vi "Main.vi"() -> ()   [LabVIEW 2015]
uses:
  TypeDefs/Queue Data.ctl
  FGV/Timer Actions.ctl
  SubVIs/App Data.vi
  SubVIs/App Strings.vi
panel:
  in  "Period [s]":dbl
  in  "Device name":tag="myDAQ1"
  out "Time Elapsed":dbl format="%<%M:%S>t"
  out "Status":string
  in  "Time [ms]":dbl
  in  "Frequency":dbl
  in  "Stop Button":bool
  in  "Acquire Button":bool
  out "Waveform Graph":dbl[](graph)
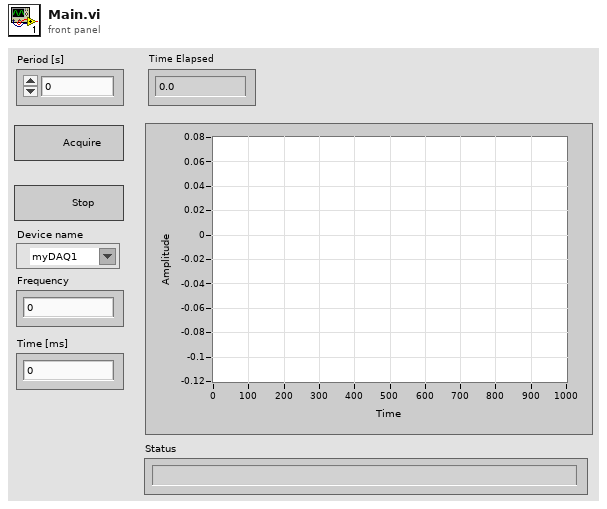
[diagram p1: front panel]
types:
  T1 = typedef "Timer Actions.ctl" = enum16{"Reset", "Get"}
  T2 = typedef "Queue Data.ctl" = cluster{"Action":string}
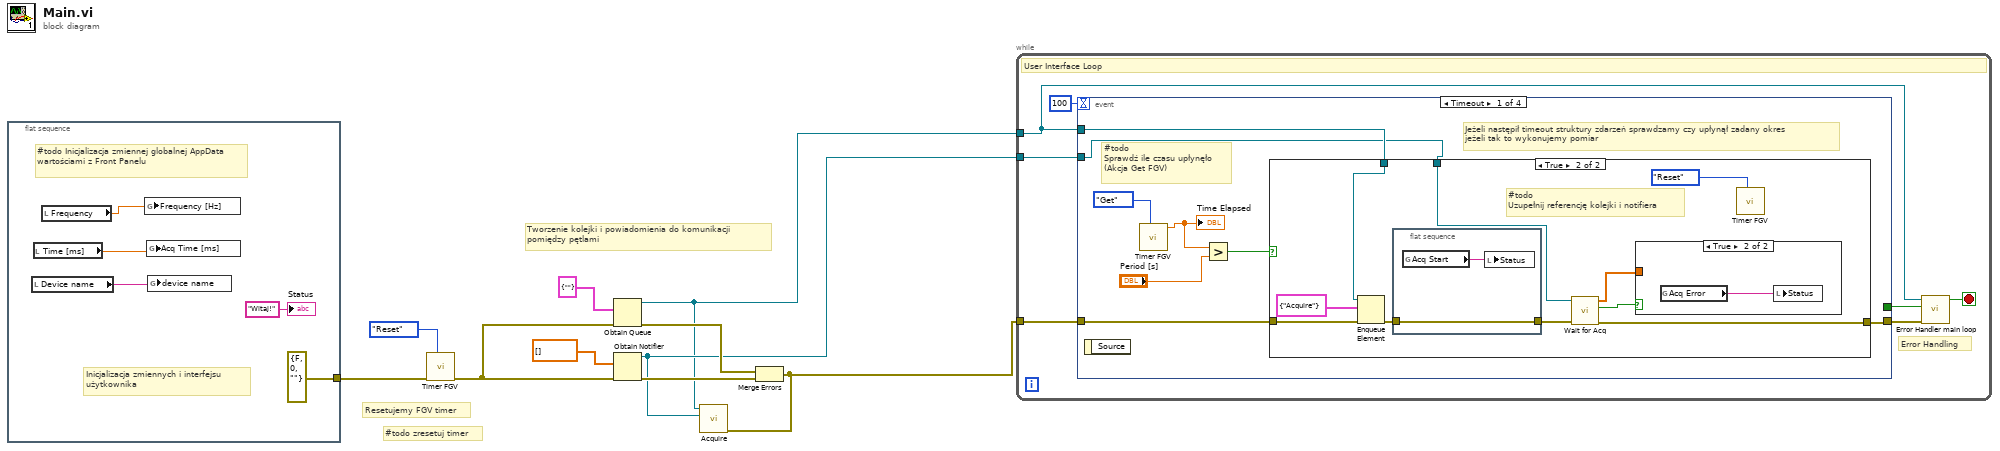
[diagram p0: block diagram]
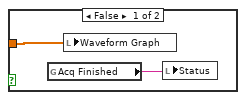
[diagram p3: hidden frame]
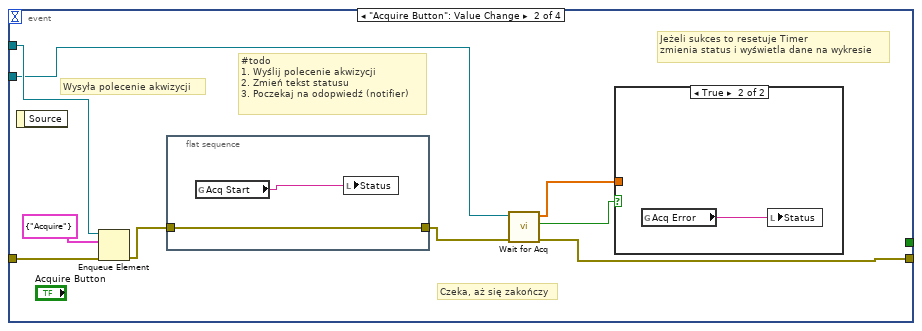
[diagram p4: hidden frame]
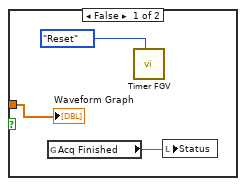
[diagram p5: hidden frame]
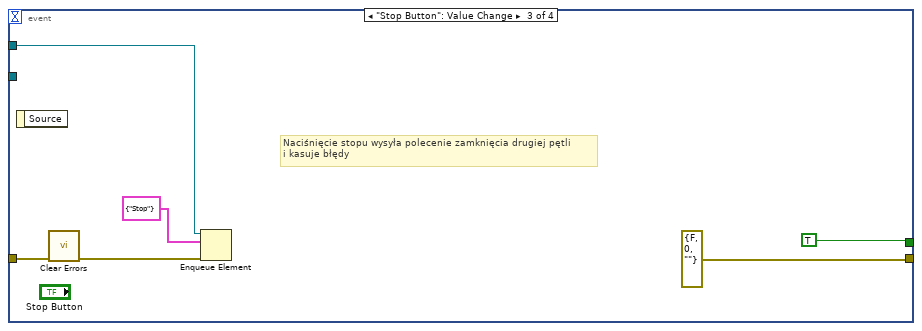
[diagram p6: hidden frame]
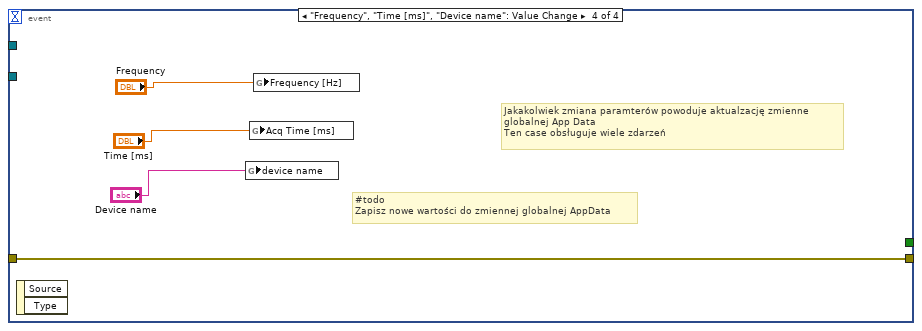
[diagram p7: hidden frame]
diagram:
  # "#todo zresetuj timer"
  # "Resetujemy FGV timer"
  # "Tworzenie kolejki i powiadomienia do komunikacji \npomiędzy pętlami"
  n1 = flat-sequence {
    tunnel: [errorcluster {"status"=FALSE, "code"=0, "source"=""} ("error constant")] -> w3
    frame #0 {
      # "#todo Inicjalizacja zmiennej globalnej AppData wartościami z Front Panelu"
      # "Inicjalizacja zmiennych i interfejsu \nużytkownika"
      n2 = local read "Device name"() -> (w11:tag)
      n3 = local read "Time [ms]"() -> (w12:dbl)
      n4 = local read "Frequency"() -> (w13:dbl)
      n5 = global write "App Data.vi" "Frequency [Hz]"(w13) -> ()
      n6 = global write "App Data.vi" "Acq Time [ms]"(w12) -> ()
      n7 = global write "App Data.vi" "device name"(w11) -> ()
      "Status" <- "Witaj!" ("Status")
    }
  }
  n8 = call "Timer FGV.vi"("Action"=Timer_Actions."Reset", "error in (no error)"=w3) -> ("error out"=w2:errorcluster)  [unwired: 8 in, 1 out]
  n9 = Obtain Queue(element data type=T2 {"Action"=""}, error in (no error)=w2) -> (queue out=w4:refnum<queue>, error out=w9:errorcluster)  [unwired: 3 in, 1 out]
  n10 = Obtain Notifier(notification data type=dbl[] [], error in (no error)=w2) -> (notifier out=w5:refnum<notifier>, error out=w7:errorcluster)  [unwired: 2 in, 1 out]
  n11 = Merge Errors(w9, w7) -> (w6:errorcluster)
  n12 = call "Acquire .vi"("error in (no error)"=w6, "notifier in"=w5, "Queue in"=w4) -> ()  [unwired: 9 in]
  n13 = while {
    tunnel: w6 -> [w21]
    tunnel: w4 -> [w17]
    tunnel: w5 -> [w16]
    stop <- w18 stop-if-true
    # "Error Handling"
    # "User Interface Loop"
    n14 = event shown="[0] Timeout" {
      selector: _ -> [_ _ _ _]
      dyn-events: _ -> [_ _ _ _]
      timeout: 100 -> [_ _ _ _]
      tunnel: w21 -> [w28 w55 w64 w71]
      tunnel: [w27 w47 errorcluster {"status"=FALSE, "code"=0, "source"=""} ("error constant") w71] -> w19
      tunnel: [_ _ TRUE _] -> w20
      tunnel: w17 -> [w24 w54 w62 _]
      tunnel: w16 -> [w23 w50 _ _]
      event Timeout {
        # "#todo\nSprawdź ile czasu upłynęło\n(Akcja Get FGV)"
        # "Jeżeli następił timeout struktury zdarzeń sprawdzamy czy upłynął zadany okres \njeżeli tak to wykonujemy pomiar"
        n15 = event-data() -> ()  [unwired: 1 in, 1 out]
        n16 = call "Timer FGV.vi"("Action"=Timer_Actions."Get") -> ("Elapsed Time"=w25:dbl)  [unwired: 9 in, 1 out]
        "Time Elapsed" <- w25
        n17 = Greater?(x=w25, y="Period [s]") -> (0:w29:bool)
        n18 = case shown="True" w29 {
          tunnel: w28 -> [w31 w41]
          tunnel: [w31 w34] -> w27
          tunnel: w24 -> [_ w33]
          tunnel: w23 -> [_ w32]
          frame False {
          }
          frame True {
            # "#todo\nUzupełnij referencję kolejki i notifiera"
            n19 = Enqueue Element(queue=w33, element=T2 {"Action"="Acquire"}, error in (no error)=w41) -> (error out=w39:errorcluster)  [unwired: 1 in, 2 out]
            n20 = flat-sequence {
              tunnel: w39 -> [w45]
              tunnel: [w45] -> w38
              frame #0 {
                n21 = global read "App Strings.vi" "Acq Start"() -> (w46:string)
                n22 = local write "Status"(w46) -> ()
              }
            }
            n23 = call "Wait for Acq.vi"("error in (no error)"=w38, "Notifier in"=w32) -> ("error out"=w34:errorcluster, "timed out?"=w35:bool, "Array"=w37:dbl[])  [unwired: 7 in]
            n24 = case shown="True" w35 {
              tunnel: w37 -> [w42 _]
              frame False {
                n25 = global read "App Strings.vi" "Acq Finished"() -> (w43:string)
                n26 = local write "Waveform Graph"(w42) -> ()
                n27 = local write "Status"(w43) -> ()
              }
              frame True {
                n28 = global read "App Strings.vi" "Acq Error"() -> (w44:string)
                n29 = local write "Status"(w44) -> ()
              }
            }
            n30 = call "Timer FGV.vi"("Action"=Timer_Actions."Reset") -> ()  [unwired: 9 in, 2 out]
          }
        }
      }
      event "Acquire Button": Value Change {
        # "#todo\n1. Wyślij polecenie akwizycji\n2. Zmień tekst statusu\n3. Poczekaj na odopwiedź (notifier)"
        # "Jeżeli sukces to resetuje Timer\nzmienia status i wyświetla dane na wykresie"
        # "Czeka, aż się zakończy"
        # "Wysyła polecenie akwizycji"
        n31 = event-data() -> ()  [unwired: 1 in, 1 out]
        n32 = Enqueue Element(queue=w54, element=T2 {"Action"="Acquire"}, error in (no error)=w55) -> (error out=w52:errorcluster)  [unwired: 1 in, 2 out]
        n33 = flat-sequence {
          tunnel: w52 -> [w56]
          tunnel: [w56] -> w51
          frame #0 {
            n34 = global read "App Strings.vi" "Acq Start"() -> (w57:string)
            n35 = local write "Status"(w57) -> ()
          }
        }
        n36 = call "Wait for Acq.vi"("error in (no error)"=w51, "Notifier in"=w50) -> ("error out"=w47:errorcluster, "timed out?"=w48:bool, "Array"=w49:dbl[])  [unwired: 7 in]
        n37 = case shown="True" w48 {
          tunnel: w49 -> [w58 _]
          frame False {
            n38 = global read "App Strings.vi" "Acq Finished"() -> (w60:string)
            n39 = call "Timer FGV.vi"("Action"=Timer_Actions."Reset") -> ()  [unwired: 9 in, 2 out]
            n40 = local write "Status"(w60) -> ()
            "Waveform Graph" <- w58
          }
          frame True {
            n41 = global read "App Strings.vi" "Acq Error"() -> (w61:string)
            n42 = local write "Status"(w61) -> ()
          }
        }
      }
      event "Stop Button": Value Change {
        # "Naciśnięcie stopu wysyła polecenie zamknięcia drugiej pętli\ni kasuje błędy"
        n43 = event-data() -> ()  [unwired: 1 in, 1 out]
        n44 = call <vilib>:"Clear Errors.vi"("error in (no error)"=w64) -> ("error out"=w63:errorcluster)  [unwired: 5 in, 1 out]
        n45 = Enqueue Element(queue=w62, element=T2 {"Action"="Stop"}, error in (no error)=w63) -> ()  [unwired: 1 in, 3 out]
      }
      event "Frequency", "Time [ms]", "Device name": Value Change {
        # "#todo \nZapisz nowe wartości do zmiennej globalnej AppData"
        # "Jakakolwiek zmiana paramterów powoduje aktualzację zmienne \nglobalnej App Data\nTen case obsługuje wiele zdarzeń"
        n46 = event-data() -> ()  [unwired: 1 in, 2 out]
        n47 = global write "App Data.vi" "device name"("Device name") -> ()
        n48 = global write "App Data.vi" "Acq Time [ms]"("Time [ms]") -> ()
        n49 = global write "App Data.vi" "Frequency [Hz]"("Frequency") -> ()
      }
    }
    n50 = call "Error Handler main loop.vi"("error in (no error)"=w19, "Exit?"=w20, "Queue in"=w17) -> ("Exit?"=w18:bool)  [unwired: 8 in]
  }
